vi "Set Oven Type.vi"(8 "Error In":errorcluster, 10 "Type":string(combo), 11 "reference in":refnum<class "Recipe Step.lvclass">) -> (0 "Error Out":errorcluster, 3 "reference out":refnum<class "Recipe Step.lvclass">)   [LabVIEW 2021, in "Recipe Step.lvclass"]
uses:
  Recipe Step.lvclass
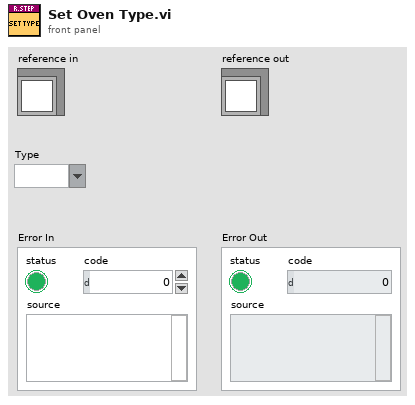
[diagram p1: front panel]
types:
  T1 = typedef "Recipe Step.lvclass/ObjectAttributes.ctl" = cluster{"Step Data":cluster{"Fire (%)":dbl, "Duration (s)":dbl, "Oven Type":string}}
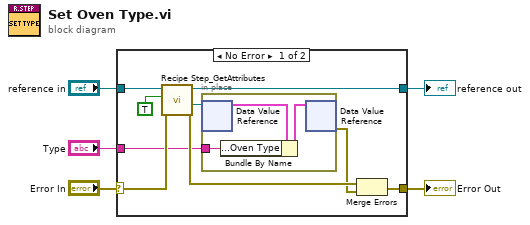
[diagram p0: block diagram]
diagram:
  n1 = case shown="No Error" "Error In" {
    selector: "Error In" -> [w13 w19]
    tunnel: [w14 w19] -> w4
    tunnel: [w10 w18] -> w2
    tunnel: "reference in" -> [w11 w18]
    tunnel: "Type" -> [w7 _]
    frame No Error {
      n2 = call "Recipe Step_GetAttributes.vi"("Error In"=w13, "OnlyGetDvrReference(False)"=TRUE, "reference in"=w11) -> ("Error Out"=w12:errorcluster, "DataRef"=w8:refnum<data-value>, "reference out"=w10:refnum<class "Recipe Step.lvclass">)  [unwired: 5 in, 1 out]
      n3 = in-place {
        in-place-border: w7 -> [w17]
        n4 = in-place-dvr #1(w8) -> (w16:T1)  [unwired: 1 out]
        n5 = Bundle By Name(cluster=w16, "Step Data.Oven Type"=w17) -> (w15:T1)
        n6 = in-place-dvr #1(w15) -> (w6:errorcluster)  [unwired: 1 out]
      }
      n7 = Merge Errors(w12, w6) -> (w14:errorcluster)
    }
    frame Error {
    }
  }
  "Error Out" <- w4
  "reference out" <- w2
